vi "Test Deserialize Strings.vi"(8 "error in (no error)":errorcluster) -> (0 "error out":errorcluster)   [LabVIEW 2013]
uses:
  src/Serializer/JSON Serializer/JSON Serializer.lvclass
  src/Deserializer/JSON Deserializer/JSON Deserializer.lvclass
  <vilib>/addons/_JKI Toolkits/Caraya/classes/Test/Test.lvclass
  <vilib>/addons/_JKI Toolkits/Caraya/classes/Assert/Assert.lvclass
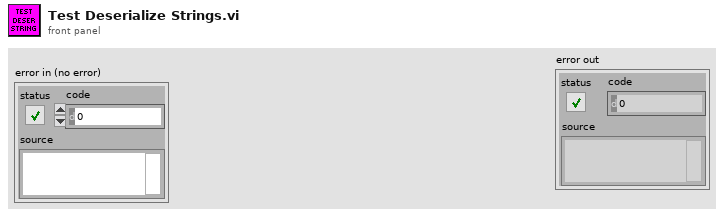
[diagram p1: front panel]
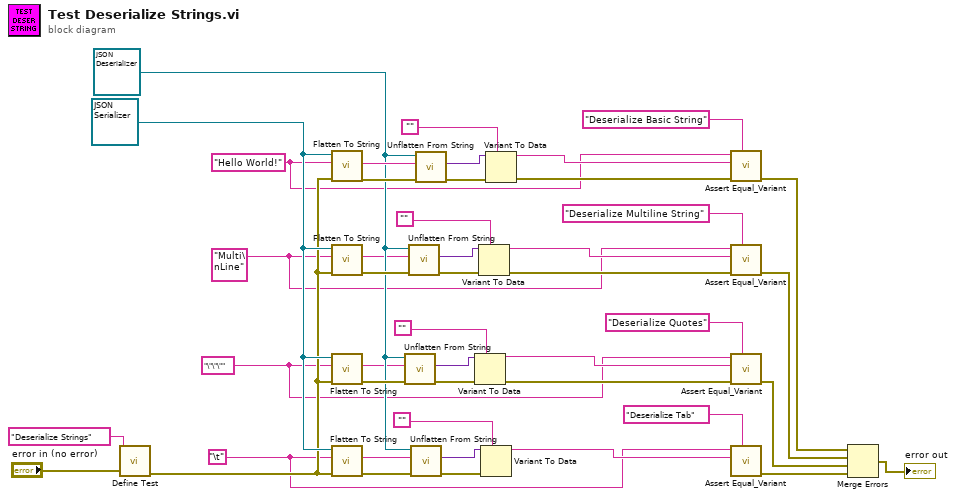
[diagram p0: block diagram]
diagram:
  w2 = "\t"
  w17 = refnum<class "JSON Deserializer.lvclass"> refnum ("Deserializer in")
  w40 = refnum<class "JSON Serializer.lvclass"> refnum ("JKI JSON Serialization.lvlib:JSON Serializer.lvclass")
  w3 = "Hello World!"
  w5 = "\"\"\""
  w4 = "Multi\nLine"
  n1 = call <vilib>:"Define Test.vi"("error in (no error)"="error in (no error)", "Label (VI Title)"="Deserialize Strings") -> ("error out"=w39:errorcluster)  [unwired: 9 in]
  n2 = call-dynamic "Flatten To String.vi"("error in (no error)"=w39, "Variant"=w3, "JSON Serializer in"=w40) -> ("error out"=w32:errorcluster, "String"=w31:string)  [unwired: 6 in, 1 out]
  n3 = call-dynamic "Flatten To String.vi"("error in (no error)"=w39, "Variant"=w4, "JSON Serializer in"=w40) -> ("error out"=w18:errorcluster, "String"=w14:string)  [unwired: 6 in, 1 out]
  n4 = call-dynamic "Flatten To String.vi"("error in (no error)"=w39, "Variant"=w5, "JSON Serializer in"=w40) -> ("error out"=w19:errorcluster, "String"=w16:string)  [unwired: 6 in, 1 out]
  n5 = call-dynamic "Flatten To String.vi"("error in (no error)"=w39, "Variant"=w2, "JSON Serializer in"=w40) -> ("error out"=w20:errorcluster, "String"=w15:string)  [unwired: 6 in, 1 out]
  n6 = call-dynamic "Unflatten From String.vi"("error in (no error)"=w19, "String"=w16, "Deserializer in"=w17) -> ("error out"=w22:errorcluster, "Variant"=w21:variant)  [unwired: 6 in, 1 out]
  n7 = call-dynamic "Unflatten From String.vi"("error in (no error)"=w18, "String"=w14, "Deserializer in"=w17) -> ("error out"=w26:errorcluster, "Variant"=w25:variant)  [unwired: 6 in, 1 out]
  n8 = call-dynamic "Unflatten From String.vi"("error in (no error)"=w20, "String"=w15, "Deserializer in"=w17) -> ("error out"=w24:errorcluster, "Variant"=w23:variant)  [unwired: 6 in, 1 out]
  n9 = call-dynamic "Unflatten From String.vi"("error in (no error)"=w32, "String"=w31, "Deserializer in"=w17) -> ("error out"=w30:errorcluster, "Variant"=w29:variant)  [unwired: 6 in, 1 out]
  n10 = Variant To Data(error in=w22, type="", Variant=w21) -> (data=w11:string, error out=w12:errorcluster)
  n11 = Variant To Data(error in=w26, type="", Variant=w25) -> (data=w9:string, error out=w13:errorcluster)
  n12 = Variant To Data(error in=w24, type="", Variant=w23) -> (data=w10:string)  [unwired: 1 out]
  n13 = Variant To Data(error in=w30, type="", Variant=w29) -> (data=w28:string, error out=w27:errorcluster)
  n14 = call <vilib>:"Assert Equal_Variant.vi"("Label"="Deserialize Basic String", "error in (no error)"=w27, "Y"=w28, "X"=w3) -> ("error out"=w34:errorcluster)  [unwired: 7 in]
  n15 = call <vilib>:"Assert Equal_Variant.vi"("Label"="Deserialize Multiline String", "error in (no error)"=w13, "Y"=w9, "X"=w4) -> ("error out"=w35:errorcluster)  [unwired: 7 in]
  n16 = call <vilib>:"Assert Equal_Variant.vi"("Label"="Deserialize Quotes", "error in (no error)"=w12, "Y"=w11, "X"=w5) -> ("error out"=w36:errorcluster)  [unwired: 7 in]
  n17 = call <vilib>:"Assert Equal_Variant.vi"("Label"="Deserialize Tab", "Y"=w10, "X"=w2) -> ("error out"=w37:errorcluster)  [unwired: 8 in]
  n18 = Merge Errors(w34, w35, w36, w37) -> (→"error out":errorcluster)
